vi "RtdeGetLatestOutputValues.vi"(8 "Rtde":refnum<k24>, 11 "error in":errorcluster) -> (0 "Data":T1, 3 "error out":errorcluster)   [LabVIEW 2022 SP3, in "UnderAutomation.UniversalRobots.lvlib"]
uses:
  UnderAutomation.UniversalRobots.lvlib
  C:/Users/fg/Documents/UniversalRobots.vi/LabVIEW_2023/UnderAutomation.UniversalRobots/lib/UnderAutomation.UniversalRobots.dll
  LabVIEW_2023/UnderAutomation.UniversalRobots/lib/UnderAutomation.UniversalRobots.dll
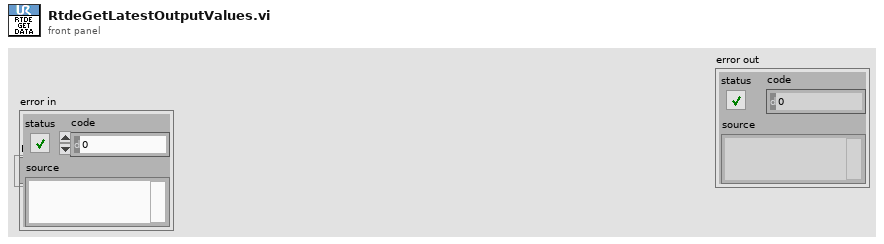
[diagram p1: front panel]
types:
  T1 = cluster{"ActualCurrent":cluster{"Base":dbl, "Elbow":dbl, "Shoulder":dbl, "Wrist1":dbl, "Wrist2":dbl, "Wrist3":dbl}, "ActualDigitalInputBits":u64, "ActualDigitalOutputBits":u64, "ActualExecutionTime":dbl, "ActualJointVoltage":cluster{"Base":dbl, "Elbow":dbl, "Shoulder":dbl, "Wrist1":dbl, "Wrist2":dbl, "Wrist3":dbl}, "ActualMainVoltage":dbl, "ActualMomentum":dbl, "ActualQ":cluster{"Base":dbl, "Elbow":dbl, "Shoulder":dbl, "Wrist1":dbl, "Wrist2":dbl, "Wrist3":dbl}, "ActualQd":cluster{"Base":dbl, "Elbow":dbl, "Shoulder":dbl, "Wrist1":dbl, "Wrist2":dbl, "Wrist3":dbl}, "ActualRobotCurrent":dbl, "ActualRobotVoltage":dbl, "ActualTcpForce":cluster{"X":dbl, "Y":dbl, "Z":dbl, "Rx":dbl, "Ry":dbl, "Rz":dbl}, "ActualTcpPose":cluster{"X":dbl, "Y":dbl, "Z":dbl, "Rx":dbl, "Ry":dbl, "Rz":dbl}, "ActualTcpSpeed":cluster{"X":dbl, "Y":dbl, "Z":dbl, "Rx":dbl, "Ry":dbl, "Rz":dbl}, "ActualToolAccelerometer":cluster{"X":dbl, "Y":dbl, "Z":dbl}, "AnalogIOTypes":u32, "ElbowPosition":cluster{"X":dbl, "Y":dbl, "Z":dbl}, "ElbowVelocity":cluster{"X":dbl, "Y":dbl, "Z":dbl}, "Euromap67_24VCurrent":dbl, "Euromap67_24VVoltage":dbl, "Euromap67InputBits":u32, "Euromap67OutputBits":u32, "FTRawWrench":cluster{"X":dbl, "Y":dbl, "Z":dbl, "Rx":dbl, "Ry":dbl, "Rz":dbl}, "InputBitRegisters":cluster{"X64":bool, "X65":bool, "X66":bool, "X67":bool, "X68":bool, "X69":bool, "X70":bool, "X71":bool, "X72":bool, "X73":bool, "X74":bool, "X75":bool, "X76":bool, "X77":bool, "X78":bool, "X79":bool, "X80":bool, "X81":bool, "X82":bool, "X83":bool, "X84":bool, "X85":bool, "X86":bool, "X87":bool, "X88":bool, "X89":bool, "X90":bool, "X91":bool, "X92":bool, "X93":bool, "X94":bool, "X95":bool, "X96":bool, "X97":bool, "X98":bool, "X99":bool, "X100":bool, "X101":bool, "X102":bool, "X103":bool, "X104":bool, "X105":bool, "X106":bool, "X107":bool, "X108":bool, "X109":bool, "X110":bool, "X111":bool, "X112":bool, "X113":bool, "X114":bool, "X115":bool, "X116":bool, "X117":bool, "X118":bool, "X119":bool, "X120":bool, "X121":bool, "X122":bool, "X123":bool, "X124":bool, "X125":bool, "X126":bool, "X127":bool}, "InputBitRegisters0To31":u32, "InputBitRegisters32To63":u32, "InputDoubleRegisters":cluster{"X0":dbl, "X1":dbl, "X2":dbl, "X3":dbl, "X4":dbl, "X5":dbl, "X6":dbl, "X7":dbl, "X8":dbl, "X9":dbl, "X10":dbl, "X11":dbl, "X12":dbl, "X13":dbl, "X14":dbl, "X15":dbl, "X16":dbl, "X17":dbl, "X18":dbl, "X19":dbl, "X20":dbl, "X21":dbl, "X22":dbl, "X23":dbl, "X24":dbl, "X25":dbl, "X26":dbl, "X27":dbl, "X28":dbl, "X29":dbl, "X30":dbl, "X31":dbl, "X32":dbl, "X33":dbl, "X34":dbl, "X35":dbl, "X36":dbl, "X37":dbl, "X38":dbl, "X39":dbl, "X40":dbl, "X41":dbl, "X42":dbl, "X43":dbl, "X44":dbl, "X45":dbl, "X46":dbl, "X47":dbl}, "InputIntRegisters":cluster{"X0":i32, "X1":i32, "X2":i32, "X3":i32, "X4":i32, "X5":i32, "X6":i32, "X7":i32, "X8":i32, "X9":i32, "X10":i32, "X11":i32, "X12":i32, "X13":i32, "X14":i32, "X15":i32, "X16":i32, "X17":i32, "X18":i32, "X19":i32, "X20":i32, "X21":i32, "X22":i32, "X23":i32, "X24":i32, "X25":i32, "X26":i32, "X27":i32, "X28":i32, "X29":i32, "X30":i32, "X31":i32, "X32":i32, "X33":i32, "X34":i32, "X35":i32, "X36":i32, "X37":i32, "X38":i32, "X39":i32, "X40":i32, "X41":i32, "X42":i32, "X43":i32, "X44":i32, "X45":i32, "X46":i32, "X47":i32}, "IOCurrent":dbl, "JointControlOutput":cluster{"Base":dbl, "Elbow":dbl, "Shoulder":dbl, "Wrist1":dbl, "Wrist2":dbl, "Wrist3":dbl}, "JointMode":cluster{"Base":i32, "Elbow":i32, "Shoulder":i32, "Wrist1":i32, "Wrist2":i32, "Wrist3":i32}, "JointTemperatures":cluster{"Base":dbl, "Elbow":dbl, "Shoulder":dbl, "Wrist1":dbl, "Wrist2":dbl, "Wrist3":dbl}, "OutputBitRegisters":cluster{"X64":bool, "X65":bool, "X66":bool, "X67":bool, "X68":bool, "X69":bool, "X70":bool, "X71":bool, "X72":bool, "X73":bool, "X74":bool, "X75":bool, "X76":bool, "X77":bool, "X78":bool, "X79":bool, "X80":bool, "X81":bool, "X82":bool, "X83":bool, "X84":bool, "X85":bool, "X86":bool, "X87":bool, "X88":bool, "X89":bool, "X90":bool, "X91":bool, "X92":bool, "X93":bool, "X94":bool, "X95":bool, "X96":bool, "X97":bool, "X98":bool, "X99":bool, "X100":bool, "X101":bool, "X102":bool, "X103":bool, "X104":bool, "X105":bool, "X106":bool, "X107":bool, "X108":bool, "X109":bool, "X110":bool, "X111":bool, "X112":bool, "X113":bool, "X114":bool, "X115":bool, "X116":bool, "X117":bool, "X118":bool, "X119":bool, "X120":bool, "X121":bool, "X122":bool, "X123":bool, "X124":bool, "X125":bool, "X126":bool, "X127":bool}, "OutputBitRegisters0To31":u32, "OutputBitRegisters32To63":u32, "OutputDoubleRegisters":cluster{"X0":dbl, "X1":dbl, "X2":dbl, "X3":dbl, "X4":dbl, "X5":dbl, "X6":dbl, "X7":dbl, "X8":dbl, "X9":dbl, "X10":dbl, "X11":dbl, "X12":dbl, "X13":dbl, "X14":dbl, "X15":dbl, "X16":dbl, "X17":dbl, "X18":dbl, "X19":dbl, "X20":dbl, "X21":dbl, "X22":dbl, "X23":dbl, "X24":dbl, "X25":dbl, "X26":dbl, "X27":dbl, "X28":dbl, "X29":dbl, "X30":dbl, "X31":dbl, "X32":dbl, "X33":dbl, "X34":dbl, "X35":dbl, "X36":dbl, "X37":dbl, "X38":dbl, "X39":dbl, "X40":dbl, "X41":dbl, "X42":dbl, "X43":dbl, "X44":dbl, "X45":dbl, "X46":dbl, "X47":dbl}, "OutputIntRegisters":cluster{"X0":i32, "X1":i32, "X2":i32, "X3":i32, "X4":i32, "X5":i32, "X6":i32, "X7":i32, "X8":i32, "X9":i32, "X10":i32, "X11":i32, "X12":i32, "X13":i32, "X14":i32, "X15":i32, "X16":i32, "X17":i32, "X18":i32, "X19":i32, "X20":i32, "X21":i32, "X22":i32, "X23":i32, "X24":i32, "X25":i32, "X26":i32, "X27":i32, "X28":i32, "X29":i32, "X30":i32, "X31":i32, "X32":i32, "X33":i32, "X34":i32, "X35":i32, "X36":i32, "X37":i32, "X38":i32, "X39":i32, "X40":i32, "X41":i32, "X42":i32, "X43":i32, "X44":i32, "X45":i32, "X46":i32, "X47":i32}, "Payload":dbl, "PayloadCOG":cluster{"X":dbl, "Y":dbl, "Z":dbl}, "PayloadInertia":cluster{"X":dbl, "Y":dbl, "Z":dbl, "Rx":dbl, "Ry":dbl, "Rz":dbl}, "RobotMode":i32, "RobotStatusBits":u32, "RuntimeState":u32, "SafetyMode":i32, "SafetyStatus":i32, "SafetyStatusBits":u32, "ScriptControlLine":u32, "SpeedScaling":dbl, "StandardAnalogInput0":dbl, "StandardAnalogInput1":dbl, "StandardAnalogOutput0":dbl, "StandardAnalogOutput1":dbl, "TargetCurrent":cluster{"Base":dbl, "Elbow":dbl, "Shoulder":dbl, "Wrist1":dbl, "Wrist2":dbl, "Wrist3":dbl}, "TargetMoment":cluster{"Base":dbl, "Elbow":dbl, "Shoulder":dbl, "Wrist1":dbl, "Wrist2":dbl, "Wrist3":dbl}, "TargetQ":cluster{"Base":dbl, "Elbow":dbl, "Shoulder":dbl, "Wrist1":dbl, "Wrist2":dbl, "Wrist3":dbl}, "TargetQd":cluster{"Base":dbl, "Elbow":dbl, "Shoulder":dbl, "Wrist1":dbl, "Wrist2":dbl, "Wrist3":dbl}, "TargetQdd":cluster{"Base":dbl, "Elbow":dbl, "Shoulder":dbl, "Wrist1":dbl, "Wrist2":dbl, "Wrist3":dbl}, "TargetSpeedFraction":dbl, "TargetTcpPose":cluster{"X":dbl, "Y":dbl, "Z":dbl, "Rx":dbl, "Ry":dbl, "Rz":dbl}, "TargetTcpSpeed":cluster{"X":dbl, "Y":dbl, "Z":dbl, "Rx":dbl, "Ry":dbl, "Rz":dbl}, "TcpForceScalar":dbl, "Timestamp":dbl, "ToolAnalogInput0":dbl, "ToolAnalogInput1":dbl, "ToolAnalogInputTypes":u32, "ToolDigitalOutput0mode":u8, "ToolDigitalOutput1Mode":u8, "ToolMode":u32, "ToolOutputCurrent":dbl, "ToolOutputMode":u8, "ToolOutputVoltage":i32, "ToolTemperature":dbl}
  T2 = cluster{"Base":dbl, "Elbow":dbl, "Shoulder":dbl, "Wrist1":dbl, "Wrist2":dbl, "Wrist3":dbl}
  T3 = cluster{"X":dbl, "Y":dbl, "Z":dbl, "Rx":dbl, "Ry":dbl, "Rz":dbl}
  T4 = cluster{"X64":bool, "X65":bool, "X66":bool, "X67":bool, "X68":bool, "X69":bool, "X70":bool, "X71":bool, "X72":bool, "X73":bool, "X74":bool, "X75":bool, "X76":bool, "X77":bool, "X78":bool, "X79":bool, "X80":bool, "X81":bool, "X82":bool, "X83":bool, "X84":bool, "X85":bool, "X86":bool, "X87":bool, "X88":bool, "X89":bool, "X90":bool, "X91":bool, "X92":bool, "X93":bool, "X94":bool, "X95":bool, "X96":bool, "X97":bool, "X98":bool, "X99":bool, "X100":bool, "X101":bool, "X102":bool, "X103":bool, "X104":bool, "X105":bool, "X106":bool, "X107":bool, "X108":bool, "X109":bool, "X110":bool, "X111":bool, "X112":bool, "X113":bool, "X114":bool, "X115":bool, "X116":bool, "X117":bool, "X118":bool, "X119":bool, "X120":bool, "X121":bool, "X122":bool, "X123":bool, "X124":bool, "X125":bool, "X126":bool, "X127":bool}
  T5 = cluster{"X0":dbl, "X1":dbl, "X2":dbl, "X3":dbl, "X4":dbl, "X5":dbl, "X6":dbl, "X7":dbl, "X8":dbl, "X9":dbl, "X10":dbl, "X11":dbl, "X12":dbl, "X13":dbl, "X14":dbl, "X15":dbl, "X16":dbl, "X17":dbl, "X18":dbl, "X19":dbl, "X20":dbl, "X21":dbl, "X22":dbl, "X23":dbl, "X24":dbl, "X25":dbl, "X26":dbl, "X27":dbl, "X28":dbl, "X29":dbl, "X30":dbl, "X31":dbl, "X32":dbl, "X33":dbl, "X34":dbl, "X35":dbl, "X36":dbl, "X37":dbl, "X38":dbl, "X39":dbl, "X40":dbl, "X41":dbl, "X42":dbl, "X43":dbl, "X44":dbl, "X45":dbl, "X46":dbl, "X47":dbl}
  T6 = cluster{"Base":i32, "Elbow":i32, "Shoulder":i32, "Wrist1":i32, "Wrist2":i32, "Wrist3":i32}
  T7 = cluster{"X0":i32, "X1":i32, "X2":i32, "X3":i32, "X4":i32, "X5":i32, "X6":i32, "X7":i32, "X8":i32, "X9":i32, "X10":i32, "X11":i32, "X12":i32, "X13":i32, "X14":i32, "X15":i32, "X16":i32, "X17":i32, "X18":i32, "X19":i32, "X20":i32, "X21":i32, "X22":i32, "X23":i32, "X24":i32, "X25":i32, "X26":i32, "X27":i32, "X28":i32, "X29":i32, "X30":i32, "X31":i32, "X32":i32, "X33":i32, "X34":i32, "X35":i32, "X36":i32, "X37":i32, "X38":i32, "X39":i32, "X40":i32, "X41":i32, "X42":i32, "X43":i32, "X44":i32, "X45":i32, "X46":i32, "X47":i32}
  T8 = cluster{cluster{"Base":dbl, "Elbow":dbl, "Shoulder":dbl, "Wrist1":dbl, "Wrist2":dbl, "Wrist3":dbl}, "ActualDigitalInputBits":u64, "ActualDigitalOutputBits":u64, "ActualExecutionTime":dbl, cluster{"Base":dbl, "Elbow":dbl, "Shoulder":dbl, "Wrist1":dbl, "Wrist2":dbl, "Wrist3":dbl}, "ActualMainVoltage":dbl, "ActualMomentum":dbl, cluster{"Base":dbl, "Elbow":dbl, "Shoulder":dbl, "Wrist1":dbl, "Wrist2":dbl, "Wrist3":dbl}, cluster{"Base":dbl, "Elbow":dbl, "Shoulder":dbl, "Wrist1":dbl, "Wrist2":dbl, "Wrist3":dbl}, "ActualRobotCurrent":dbl, "ActualRobotVoltage":dbl, cluster{"X":dbl, "Y":dbl, "Z":dbl, "Rx":dbl, "Ry":dbl, "Rz":dbl}, cluster{"X":dbl, "Y":dbl, "Z":dbl, "Rx":dbl, "Ry":dbl, "Rz":dbl}, cluster{"X":dbl, "Y":dbl, "Z":dbl, "Rx":dbl, "Ry":dbl, "Rz":dbl}, cluster{"X":dbl, "Y":dbl, "Z":dbl}, "AnalogIOTypes":u32, cluster{"X":dbl, "Y":dbl, "Z":dbl}, cluster{"X":dbl, "Y":dbl, "Z":dbl}, "Euromap67_24VCurrent":dbl, "Euromap67_24VVoltage":dbl, "Euromap67InputBits":u32, "Euromap67OutputBits":u32, cluster{"X":dbl, "Y":dbl, "Z":dbl, "Rx":dbl, "Ry":dbl, "Rz":dbl}, cluster{"X64":bool, "X65":bool, "X66":bool, "X67":bool, "X68":bool, "X69":bool, "X70":bool, "X71":bool, "X72":bool, "X73":bool, "X74":bool, "X75":bool, "X76":bool, "X77":bool, "X78":bool, "X79":bool, "X80":bool, "X81":bool, "X82":bool, "X83":bool, "X84":bool, "X85":bool, "X86":bool, "X87":bool, "X88":bool, "X89":bool, "X90":bool, "X91":bool, "X92":bool, "X93":bool, "X94":bool, "X95":bool, "X96":bool, "X97":bool, "X98":bool, "X99":bool, "X100":bool, "X101":bool, "X102":bool, "X103":bool, "X104":bool, "X105":bool, "X106":bool, "X107":bool, "X108":bool, "X109":bool, "X110":bool, "X111":bool, "X112":bool, "X113":bool, "X114":bool, "X115":bool, "X116":bool, "X117":bool, "X118":bool, "X119":bool, "X120":bool, "X121":bool, "X122":bool, "X123":bool, "X124":bool, "X125":bool, "X126":bool, "X127":bool}, "InputBitRegisters0To31":u32, "InputBitRegisters32To63":u32, cluster{"X0":dbl, "X1":dbl, "X2":dbl, "X3":dbl, "X4":dbl, "X5":dbl, "X6":dbl, "X7":dbl, "X8":dbl, "X9":dbl, "X10":dbl, "X11":dbl, "X12":dbl, "X13":dbl, "X14":dbl, "X15":dbl, "X16":dbl, "X17":dbl, "X18":dbl, "X19":dbl, "X20":dbl, "X21":dbl, "X22":dbl, "X23":dbl, "X24":dbl, "X25":dbl, "X26":dbl, "X27":dbl, "X28":dbl, "X29":dbl, "X30":dbl, "X31":dbl, "X32":dbl, "X33":dbl, "X34":dbl, "X35":dbl, "X36":dbl, "X37":dbl, "X38":dbl, "X39":dbl, "X40":dbl, "X41":dbl, "X42":dbl, "X43":dbl, "X44":dbl, "X45":dbl, "X46":dbl, "X47":dbl}, cluster{"X0":i32, "X1":i32, "X2":i32, "X3":i32, "X4":i32, "X5":i32, "X6":i32, "X7":i32, "X8":i32, "X9":i32, "X10":i32, "X11":i32, "X12":i32, "X13":i32, "X14":i32, "X15":i32, "X16":i32, "X17":i32, "X18":i32, "X19":i32, "X20":i32, "X21":i32, "X22":i32, "X23":i32, "X24":i32, "X25":i32, "X26":i32, "X27":i32, "X28":i32, "X29":i32, "X30":i32, "X31":i32, "X32":i32, "X33":i32, "X34":i32, "X35":i32, "X36":i32, "X37":i32, "X38":i32, "X39":i32, "X40":i32, "X41":i32, "X42":i32, "X43":i32, "X44":i32, "X45":i32, "X46":i32, "X47":i32}, "IOCurrent":dbl, cluster{"Base":dbl, "Elbow":dbl, "Shoulder":dbl, "Wrist1":dbl, "Wrist2":dbl, "Wrist3":dbl}, cluster{"Base":i32, "Elbow":i32, "Shoulder":i32, "Wrist1":i32, "Wrist2":i32, "Wrist3":i32}, cluster{"Base":dbl, "Elbow":dbl, "Shoulder":dbl, "Wrist1":dbl, "Wrist2":dbl, "Wrist3":dbl}, cluster{"X64":bool, "X65":bool, "X66":bool, "X67":bool, "X68":bool, "X69":bool, "X70":bool, "X71":bool, "X72":bool, "X73":bool, "X74":bool, "X75":bool, "X76":bool, "X77":bool, "X78":bool, "X79":bool, "X80":bool, "X81":bool, "X82":bool, "X83":bool, "X84":bool, "X85":bool, "X86":bool, "X87":bool, "X88":bool, "X89":bool, "X90":bool, "X91":bool, "X92":bool, "X93":bool, "X94":bool, "X95":bool, "X96":bool, "X97":bool, "X98":bool, "X99":bool, "X100":bool, "X101":bool, "X102":bool, "X103":bool, "X104":bool, "X105":bool, "X106":bool, "X107":bool, "X108":bool, "X109":bool, "X110":bool, "X111":bool, "X112":bool, "X113":bool, "X114":bool, "X115":bool, "X116":bool, "X117":bool, "X118":bool, "X119":bool, "X120":bool, "X121":bool, "X122":bool, "X123":bool, "X124":bool, "X125":bool, "X126":bool, "X127":bool}, "OutputBitRegisters0To31":u32, "OutputBitRegisters32To63":u32, cluster{"X0":dbl, "X1":dbl, "X2":dbl, "X3":dbl, "X4":dbl, "X5":dbl, "X6":dbl, "X7":dbl, "X8":dbl, "X9":dbl, "X10":dbl, "X11":dbl, "X12":dbl, "X13":dbl, "X14":dbl, "X15":dbl, "X16":dbl, "X17":dbl, "X18":dbl, "X19":dbl, "X20":dbl, "X21":dbl, "X22":dbl, "X23":dbl, "X24":dbl, "X25":dbl, "X26":dbl, "X27":dbl, "X28":dbl, "X29":dbl, "X30":dbl, "X31":dbl, "X32":dbl, "X33":dbl, "X34":dbl, "X35":dbl, "X36":dbl, "X37":dbl, "X38":dbl, "X39":dbl, "X40":dbl, "X41":dbl, "X42":dbl, "X43":dbl, "X44":dbl, "X45":dbl, "X46":dbl, "X47":dbl}, cluster{"X0":i32, "X1":i32, "X2":i32, "X3":i32, "X4":i32, "X5":i32, "X6":i32, "X7":i32, "X8":i32, "X9":i32, "X10":i32, "X11":i32, "X12":i32, "X13":i32, "X14":i32, "X15":i32, "X16":i32, "X17":i32, "X18":i32, "X19":i32, "X20":i32, "X21":i32, "X22":i32, "X23":i32, "X24":i32, "X25":i32, "X26":i32, "X27":i32, "X28":i32, "X29":i32, "X30":i32, "X31":i32, "X32":i32, "X33":i32, "X34":i32, "X35":i32, "X36":i32, "X37":i32, "X38":i32, "X39":i32, "X40":i32, "X41":i32, "X42":i32, "X43":i32, "X44":i32, "X45":i32, "X46":i32, "X47":i32}, "Payload":dbl, cluster{"X":dbl, "Y":dbl, "Z":dbl}, cluster{"X":dbl, "Y":dbl, "Z":dbl, "Rx":dbl, "Ry":dbl, "Rz":dbl}, "RobotMode":i32, "RobotStatusBits":u32, "RuntimeState":u32, "SafetyMode":i32, "SafetyStatus":i32, "SafetyStatusBits":u32, "ScriptControlLine":u32, "SpeedScaling":dbl, "StandardAnalogInput0":dbl, "StandardAnalogInput1":dbl, "StandardAnalogOutput0":dbl, "StandardAnalogOutput1":dbl, cluster{"Base":dbl, "Elbow":dbl, "Shoulder":dbl, "Wrist1":dbl, "Wrist2":dbl, "Wrist3":dbl}, cluster{"Base":dbl, "Elbow":dbl, "Shoulder":dbl, "Wrist1":dbl, "Wrist2":dbl, "Wrist3":dbl}, cluster{"Base":dbl, "Elbow":dbl, "Shoulder":dbl, "Wrist1":dbl, "Wrist2":dbl, "Wrist3":dbl}, cluster{"Base":dbl, "Elbow":dbl, "Shoulder":dbl, "Wrist1":dbl, "Wrist2":dbl, "Wrist3":dbl}, cluster{"Base":dbl, "Elbow":dbl, "Shoulder":dbl, "Wrist1":dbl, "Wrist2":dbl, "Wrist3":dbl}, "TargetSpeedFraction":dbl, cluster{"X":dbl, "Y":dbl, "Z":dbl, "Rx":dbl, "Ry":dbl, "Rz":dbl}, cluster{"X":dbl, "Y":dbl, "Z":dbl, "Rx":dbl, "Ry":dbl, "Rz":dbl}, "TcpForceScalar":dbl, "Timestamp":dbl, "ToolAnalogInput0":dbl, "ToolAnalogInput1":dbl, "ToolAnalogInputTypes":u32, "ToolDigitalOutput0mode":u8, "ToolDigitalOutput1Mode":u8, "ToolMode":u32, "ToolOutputCurrent":dbl, "ToolOutputMode":u8, "ToolOutputVoltage":i32, "ToolTemperature":dbl}
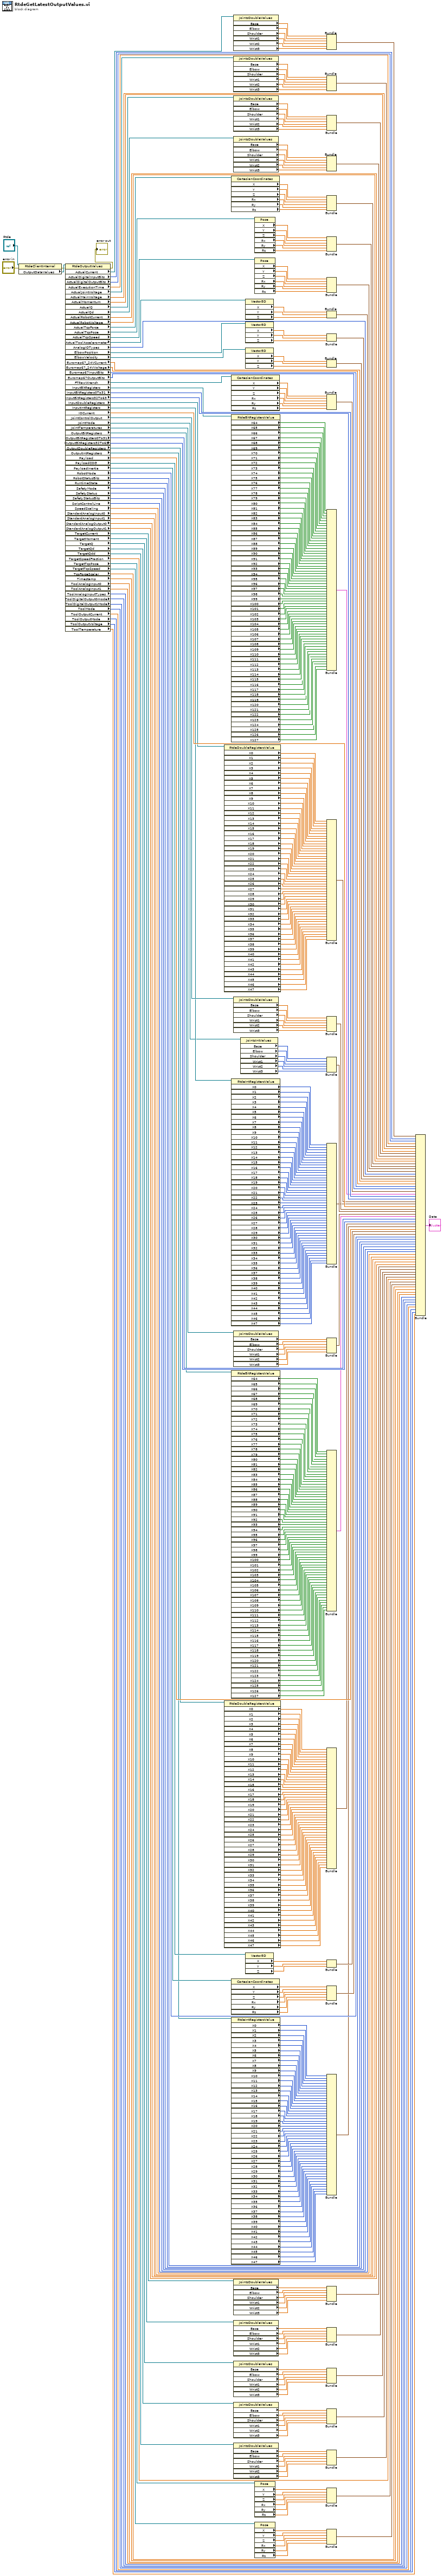
[diagram p0: block diagram]
diagram:
  n1 = property class="RtdeClientInternal"(reference="Rtde", error in="error in") -> (error out=w1:errorcluster, "OutputDataValues"=w2:refnum<k24>)  [unwired: 1 out]
  n2 = property on="Property Node" class="RtdeOutputValues"(reference=w2, error in=w1) -> (error out=→"error out":errorcluster, "ActualCurrent"=w4:refnum<k24>, "ActualDigitalInputBits"=w126:u64, "ActualDigitalOutputBits"=w127:u64, "ActualExecutionTime"=w128:dbl, "ActualJointVoltage"=w11:refnum<k24>, "ActualMainVoltage"=w130:dbl, "ActualMomentum"=w131:dbl, "ActualQ"=w83:refnum<k24>, "ActualQd"=w90:refnum<k24>, "ActualRobotCurrent"=w134:dbl, "ActualRobotVoltage"=w135:dbl, "ActualTcpForce"=w149:refnum<k24>, "ActualTcpPose"=w136:refnum<k24>, "ActualTcpSpeed"=w158:refnum<k24>, "ActualToolAccelerometer"=w160:refnum<k24>, "AnalogIOTypes"=w165:u32, "ElbowPosition"=w166:refnum<k24>, "ElbowVelocity"=w171:refnum<k24>, "Euromap67_24VCurrent"=w176:dbl, "Euromap67_24VVoltage"=w177:dbl, "Euromap67InputBits"=w178:u32, "Euromap67OutputBits"=w179:u32, "FTRawWrench"=w186:refnum<k24>, "InputBitRegisters"=w252:refnum<k24>, "InputBitRegisters0To31"=w304:u32, "InputBitRegisters32To63"=w303:u32, "InputDoubleRegisters"=w254:refnum<k24>, "InputIntRegisters"=w354:refnum<k24>, "IOCurrent"=w356:dbl, "JointControlOutput"=w363:refnum<k24>, "JointMode"=w97:refnum<k24>, "JointTemperatures"=w372:refnum<k24>, "OutputBitRegisters"=w12:refnum<k24>, "OutputBitRegisters0To31"=w375:u32, "OutputBitRegisters32To63"=w376:u32, "OutputDoubleRegisters"=w425:refnum<k24>, "OutputIntRegisters"=w475:refnum<k24>, "Payload"=w481:dbl, "PayloadCOG"=w480:refnum<k24>, "PayloadInertia"=w489:refnum<k24>, "RobotMode"=w491:i32, "RobotStatusBits"=w492:u32, "RuntimeState"=w493:u32, "SafetyMode"=w494:i32, "SafetyStatus"=w495:i32, "SafetyStatusBits"=w496:u32, "ScriptControlLine"=w497:u32, "SpeedScaling"=w498:dbl, "StandardAnalogInput0"=w499:dbl, "StandardAnalogInput1"=w500:dbl, "StandardAnalogOutput0"=w501:dbl, "StandardAnalogOutput1"=w502:dbl, "TargetCurrent"=w515:refnum<k24>, "TargetMoment"=w516:refnum<k24>, "TargetQ"=w122:refnum<k24>, "TargetQd"=w123:refnum<k24>, "TargetQdd"=w124:refnum<k24>, "TargetSpeedFraction"=w522:dbl, "TargetTcpPose"=w535:refnum<k24>, "TargetTcpSpeed"=w536:refnum<k24>, "TcpForceScalar"=w539:dbl, "Timestamp"=w540:dbl, "ToolAnalogInput0"=w541:dbl, "ToolAnalogInput1"=w542:dbl, "ToolAnalogInputTypes"=w543:u32, "ToolDigitalOutput0mode"=w544:u8, "ToolDigitalOutput1Mode"=w545:u8, "ToolMode"=w546:u32, "ToolOutputCurrent"=w547:dbl, "ToolOutputMode"=w548:u8, "ToolOutputVoltage"=w549:i32, "ToolTemperature"=w550:dbl)  [unwired: 1 out]
  n3 = property class="RtdeDoubleRegistersValue"(reference=w254) -> ("X0"=w255:dbl, "X1"=w256:dbl, "X2"=w257:dbl, "X3"=w258:dbl, "X4"=w259:dbl, "X5"=w260:dbl, "X6"=w261:dbl, "X7"=w262:dbl, "X8"=w263:dbl, "X9"=w264:dbl, "X10"=w265:dbl, "X11"=w266:dbl, "X12"=w267:dbl, "X13"=w268:dbl, "X14"=w269:dbl, "X15"=w270:dbl, "X16"=w271:dbl, "X17"=w272:dbl, "X18"=w273:dbl, "X19"=w274:dbl, "X20"=w275:dbl, "X21"=w276:dbl, "X22"=w277:dbl, "X23"=w278:dbl, "X24"=w279:dbl, "X25"=w280:dbl, "X26"=w281:dbl, "X27"=w282:dbl, "X28"=w283:dbl, "X29"=w284:dbl, "X30"=w285:dbl, "X31"=w286:dbl, "X32"=w287:dbl, "X33"=w288:dbl, "X34"=w289:dbl, "X35"=w290:dbl, "X36"=w291:dbl, "X37"=w292:dbl, "X38"=w293:dbl, "X39"=w294:dbl, "X40"=w295:dbl, "X41"=w296:dbl, "X42"=w297:dbl, "X43"=w298:dbl, "X44"=w299:dbl, "X45"=w300:dbl, "X46"=w301:dbl, "X47"=w302:dbl)  [unwired: 1 in, 2 out]
  n4 = property class="RtdeDoubleRegistersValue"(reference=w425) -> ("X0"=w377:dbl, "X1"=w378:dbl, "X2"=w379:dbl, "X3"=w380:dbl, "X4"=w381:dbl, "X5"=w382:dbl, "X6"=w383:dbl, "X7"=w384:dbl, "X8"=w385:dbl, "X9"=w386:dbl, "X10"=w387:dbl, "X11"=w388:dbl, "X12"=w389:dbl, "X13"=w390:dbl, "X14"=w391:dbl, "X15"=w392:dbl, "X16"=w393:dbl, "X17"=w394:dbl, "X18"=w395:dbl, "X19"=w396:dbl, "X20"=w397:dbl, "X21"=w398:dbl, "X22"=w399:dbl, "X23"=w400:dbl, "X24"=w401:dbl, "X25"=w402:dbl, "X26"=w403:dbl, "X27"=w404:dbl, "X28"=w405:dbl, "X29"=w406:dbl, "X30"=w407:dbl, "X31"=w408:dbl, "X32"=w409:dbl, "X33"=w410:dbl, "X34"=w411:dbl, "X35"=w412:dbl, "X36"=w413:dbl, "X37"=w414:dbl, "X38"=w415:dbl, "X39"=w416:dbl, "X40"=w417:dbl, "X41"=w418:dbl, "X42"=w419:dbl, "X43"=w420:dbl, "X44"=w421:dbl, "X45"=w422:dbl, "X46"=w423:dbl, "X47"=w424:dbl)  [unwired: 1 in, 2 out]
  n5 = property class="CartesianCoordinates"(reference=w149) -> ("X"=w148:dbl, "Y"=w147:dbl, "Z"=w146:dbl, "Rx"=w145:dbl, "Ry"=w144:dbl, "Rz"=w143:dbl)  [unwired: 1 in, 2 out]
  n6 = property class="CartesianCoordinates"(reference=w186) -> ("X"=w180:dbl, "Y"=w181:dbl, "Z"=w182:dbl, "Rx"=w183:dbl, "Ry"=w184:dbl, "Rz"=w185:dbl)  [unwired: 1 in, 2 out]
  n7 = property class="CartesianCoordinates"(reference=w489) -> ("X"=w483:dbl, "Y"=w484:dbl, "Z"=w485:dbl, "Rx"=w486:dbl, "Ry"=w487:dbl, "Rz"=w488:dbl)  [unwired: 1 in, 2 out]
  n8 = property class="RtdeBitRegistersValue"(reference=w252) -> ("X64"=w251:bool, "X65"=w250:bool, "X66"=w249:bool, "X67"=w248:bool, "X68"=w247:bool, "X69"=w246:bool, "X70"=w245:bool, "X71"=w244:bool, "X72"=w243:bool, "X73"=w242:bool, "X74"=w241:bool, "X75"=w240:bool, "X76"=w239:bool, "X77"=w238:bool, "X78"=w237:bool, "X79"=w236:bool, "X80"=w235:bool, "X81"=w234:bool, "X82"=w233:bool, "X83"=w232:bool, "X84"=w231:bool, "X85"=w230:bool, "X86"=w229:bool, "X87"=w228:bool, "X88"=w227:bool, "X89"=w226:bool, "X90"=w225:bool, "X91"=w224:bool, "X92"=w223:bool, "X93"=w222:bool, "X94"=w221:bool, "X95"=w220:bool, "X96"=w219:bool, "X97"=w218:bool, "X98"=w217:bool, "X99"=w216:bool, "X100"=w215:bool, "X101"=w214:bool, "X102"=w213:bool, "X103"=w212:bool, "X104"=w211:bool, "X105"=w210:bool, "X106"=w209:bool, "X107"=w208:bool, "X108"=w207:bool, "X109"=w206:bool, "X110"=w205:bool, "X111"=w204:bool, "X112"=w203:bool, "X113"=w202:bool, "X114"=w201:bool, "X115"=w200:bool, "X116"=w199:bool, "X117"=w198:bool, "X118"=w197:bool, "X119"=w196:bool, "X120"=w195:bool, "X121"=w194:bool, "X122"=w193:bool, "X123"=w192:bool, "X124"=w191:bool, "X125"=w190:bool, "X126"=w189:bool, "X127"=w188:bool)  [unwired: 1 in, 2 out]
  n9 = property class="RtdeIntRegistersValue"(reference=w354) -> ("X0"=w306:i32, "X1"=w307:i32, "X2"=w308:i32, "X3"=w309:i32, "X4"=w310:i32, "X5"=w311:i32, "X6"=w312:i32, "X7"=w313:i32, "X8"=w314:i32, "X9"=w315:i32, "X10"=w316:i32, "X11"=w317:i32, "X12"=w318:i32, "X13"=w319:i32, "X14"=w320:i32, "X15"=w321:i32, "X16"=w322:i32, "X17"=w323:i32, "X18"=w324:i32, "X19"=w325:i32, "X20"=w326:i32, "X21"=w327:i32, "X22"=w328:i32, "X23"=w329:i32, "X24"=w330:i32, "X25"=w331:i32, "X26"=w332:i32, "X27"=w333:i32, "X28"=w334:i32, "X29"=w335:i32, "X30"=w336:i32, "X31"=w337:i32, "X32"=w338:i32, "X33"=w339:i32, "X34"=w340:i32, "X35"=w341:i32, "X36"=w342:i32, "X37"=w343:i32, "X38"=w344:i32, "X39"=w345:i32, "X40"=w346:i32, "X41"=w347:i32, "X42"=w348:i32, "X43"=w349:i32, "X44"=w350:i32, "X45"=w351:i32, "X46"=w352:i32, "X47"=w353:i32)  [unwired: 1 in, 2 out]
  n10 = property class="RtdeBitRegistersValue"(reference=w12) -> ("X64"=w13:bool, "X65"=w14:bool, "X66"=w15:bool, "X67"=w16:bool, "X68"=w17:bool, "X69"=w18:bool, "X70"=w19:bool, "X71"=w20:bool, "X72"=w21:bool, "X73"=w22:bool, "X74"=w23:bool, "X75"=w24:bool, "X76"=w25:bool, "X77"=w26:bool, "X78"=w27:bool, "X79"=w28:bool, "X80"=w29:bool, "X81"=w30:bool, "X82"=w31:bool, "X83"=w32:bool, "X84"=w33:bool, "X85"=w34:bool, "X86"=w35:bool, "X87"=w36:bool, "X88"=w37:bool, "X89"=w38:bool, "X90"=w39:bool, "X91"=w40:bool, "X92"=w41:bool, "X93"=w42:bool, "X94"=w43:bool, "X95"=w44:bool, "X96"=w45:bool, "X97"=w46:bool, "X98"=w47:bool, "X99"=w48:bool, "X100"=w49:bool, "X101"=w50:bool, "X102"=w51:bool, "X103"=w52:bool, "X104"=w53:bool, "X105"=w54:bool, "X106"=w55:bool, "X107"=w56:bool, "X108"=w57:bool, "X109"=w58:bool, "X110"=w59:bool, "X111"=w60:bool, "X112"=w61:bool, "X113"=w62:bool, "X114"=w63:bool, "X115"=w64:bool, "X116"=w65:bool, "X117"=w66:bool, "X118"=w67:bool, "X119"=w68:bool, "X120"=w69:bool, "X121"=w70:bool, "X122"=w71:bool, "X123"=w72:bool, "X124"=w73:bool, "X125"=w74:bool, "X126"=w75:bool, "X127"=w76:bool)  [unwired: 1 in, 2 out]
  n11 = property class="RtdeIntRegistersValue"(reference=w475) -> ("X0"=w474:i32, "X1"=w473:i32, "X2"=w472:i32, "X3"=w471:i32, "X4"=w470:i32, "X5"=w469:i32, "X6"=w468:i32, "X7"=w467:i32, "X8"=w466:i32, "X9"=w465:i32, "X10"=w464:i32, "X11"=w463:i32, "X12"=w462:i32, "X13"=w461:i32, "X14"=w460:i32, "X15"=w459:i32, "X16"=w458:i32, "X17"=w457:i32, "X18"=w456:i32, "X19"=w455:i32, "X20"=w454:i32, "X21"=w453:i32, "X22"=w452:i32, "X23"=w451:i32, "X24"=w450:i32, "X25"=w449:i32, "X26"=w448:i32, "X27"=w447:i32, "X28"=w446:i32, "X29"=w445:i32, "X30"=w444:i32, "X31"=w443:i32, "X32"=w442:i32, "X33"=w441:i32, "X34"=w440:i32, "X35"=w439:i32, "X36"=w438:i32, "X37"=w437:i32, "X38"=w436:i32, "X39"=w435:i32, "X40"=w434:i32, "X41"=w433:i32, "X42"=w432:i32, "X43"=w431:i32, "X44"=w430:i32, "X45"=w429:i32, "X46"=w428:i32, "X47"=w427:i32)  [unwired: 1 in, 2 out]
  n12 = property class="JointsDoubleValues"(reference=w4) -> ("Base"=w5:dbl, "Elbow"=w6:dbl, "Shoulder"=w7:dbl, "Wrist1"=w8:dbl, "Wrist2"=w9:dbl, "Wrist3"=w10:dbl)  [unwired: 1 in, 2 out]
  n13 = property class="JointsDoubleValues"(reference=w11) -> ("Base"=w91:dbl, "Elbow"=w92:dbl, "Shoulder"=w93:dbl, "Wrist1"=w94:dbl, "Wrist2"=w95:dbl, "Wrist3"=w96:dbl)  [unwired: 1 in, 2 out]
  n14 = property class="JointsDoubleValues"(reference=w83) -> ("Base"=w77:dbl, "Elbow"=w78:dbl, "Shoulder"=w79:dbl, "Wrist1"=w80:dbl, "Wrist2"=w81:dbl, "Wrist3"=w82:dbl)  [unwired: 1 in, 2 out]
  n15 = property class="JointsDoubleValues"(reference=w90) -> ("Base"=w84:dbl, "Elbow"=w85:dbl, "Shoulder"=w86:dbl, "Wrist1"=w87:dbl, "Wrist2"=w88:dbl, "Wrist3"=w89:dbl)  [unwired: 1 in, 2 out]
  n16 = property class="JointsDoubleValues"(reference=w363) -> ("Base"=w357:dbl, "Elbow"=w358:dbl, "Shoulder"=w359:dbl, "Wrist1"=w360:dbl, "Wrist2"=w361:dbl, "Wrist3"=w362:dbl)  [unwired: 1 in, 2 out]
  n17 = property class="JointsDoubleValues"(reference=w372) -> ("Base"=w371:dbl, "Elbow"=w370:dbl, "Shoulder"=w369:dbl, "Wrist1"=w368:dbl, "Wrist2"=w367:dbl, "Wrist3"=w366:dbl)  [unwired: 1 in, 2 out]
  n18 = property class="JointsDoubleValues"(reference=w515) -> ("Base"=w509:dbl, "Elbow"=w510:dbl, "Shoulder"=w511:dbl, "Wrist1"=w512:dbl, "Wrist2"=w513:dbl, "Wrist3"=w514:dbl)  [unwired: 1 in, 2 out]
  n19 = property class="JointsDoubleValues"(reference=w516) -> ("Base"=w508:dbl, "Elbow"=w507:dbl, "Shoulder"=w506:dbl, "Wrist1"=w505:dbl, "Wrist2"=w504:dbl, "Wrist3"=w503:dbl)  [unwired: 1 in, 2 out]
  n20 = property class="JointsDoubleValues"(reference=w122) -> ("Base"=w104:dbl, "Elbow"=w105:dbl, "Shoulder"=w106:dbl, "Wrist1"=w107:dbl, "Wrist2"=w108:dbl, "Wrist3"=w109:dbl)  [unwired: 1 in, 2 out]
  n21 = property class="JointsDoubleValues"(reference=w123) -> ("Base"=w110:dbl, "Elbow"=w111:dbl, "Shoulder"=w112:dbl, "Wrist1"=w113:dbl, "Wrist2"=w114:dbl, "Wrist3"=w115:dbl)  [unwired: 1 in, 2 out]
  n22 = property class="JointsDoubleValues"(reference=w124) -> ("Base"=w116:dbl, "Elbow"=w117:dbl, "Shoulder"=w118:dbl, "Wrist1"=w119:dbl, "Wrist2"=w120:dbl, "Wrist3"=w121:dbl)  [unwired: 1 in, 2 out]
  n23 = property class="JointsIntValues"(reference=w97) -> ("Base"=w98:i32, "Elbow"=w99:i32, "Shoulder"=w100:i32, "Wrist1"=w101:i32, "Wrist2"=w102:i32, "Wrist3"=w103:i32)  [unwired: 1 in, 2 out]
  n24 = property class="Vector3D"(reference=w160) -> ("X"=w161:dbl, "Y"=w162:dbl, "Z"=w163:dbl)  [unwired: 1 in, 2 out]
  n25 = property class="Vector3D"(reference=w166) -> ("X"=w167:dbl, "Y"=w168:dbl, "Z"=w169:dbl)  [unwired: 1 in, 2 out]
  n26 = property class="Vector3D"(reference=w171) -> ("X"=w172:dbl, "Y"=w173:dbl, "Z"=w174:dbl)  [unwired: 1 in, 2 out]
  n27 = property class="Vector3D"(reference=w480) -> ("X"=w477:dbl, "Y"=w478:dbl, "Z"=w479:dbl)  [unwired: 1 in, 2 out]
  n28 = property class="Pose"(reference=w136) -> ("X"=w137:dbl, "Y"=w138:dbl, "Z"=w139:dbl, "Rx"=w140:dbl, "Ry"=w141:dbl, "Rz"=w142:dbl)  [unwired: 1 in, 2 out]
  n29 = property class="Pose"(reference=w158) -> ("X"=w152:dbl, "Y"=w153:dbl, "Z"=w154:dbl, "Rx"=w155:dbl, "Ry"=w156:dbl, "Rz"=w157:dbl)  [unwired: 1 in, 2 out]
  n30 = property class="Pose"(reference=w535) -> ("X"=w523:dbl, "Y"=w524:dbl, "Z"=w525:dbl, "Rx"=w526:dbl, "Ry"=w527:dbl, "Rz"=w528:dbl)  [unwired: 1 in, 2 out]
  n31 = property class="Pose"(reference=w536) -> ("X"=w529:dbl, "Y"=w530:dbl, "Z"=w531:dbl, "Rx"=w532:dbl, "Ry"=w533:dbl, "Rz"=w534:dbl)  [unwired: 1 in, 2 out]
  n32 = Bundle("Base"=w5, "Elbow"=w6, "Shoulder"=w7, "Wrist1"=w8, "Wrist2"=w9, "Wrist3"=w10) -> (w125:T2)  [unwired: 1 in]
  n33 = Bundle("Base"=w91, "Elbow"=w92, "Shoulder"=w93, "Wrist1"=w94, "Wrist2"=w95, "Wrist3"=w96) -> (w129:T2)  [unwired: 1 in]
  n34 = Bundle("Base"=w77, "Elbow"=w78, "Shoulder"=w79, "Wrist1"=w80, "Wrist2"=w81, "Wrist3"=w82) -> (w132:T2)  [unwired: 1 in]
  n35 = Bundle("Base"=w84, "Elbow"=w85, "Shoulder"=w86, "Wrist1"=w87, "Wrist2"=w88, "Wrist3"=w89) -> (w133:T2)  [unwired: 1 in]
  n36 = Bundle("X"=w148, "Y"=w147, "Z"=w146, "Rx"=w145, "Ry"=w144, "Rz"=w143) -> (w150:T3)  [unwired: 1 in]
  n37 = Bundle("X"=w137, "Y"=w138, "Z"=w139, "Rx"=w140, "Ry"=w141, "Rz"=w142) -> (w151:T3)  [unwired: 1 in]
  n38 = Bundle("X"=w152, "Y"=w153, "Z"=w154, "Rx"=w155, "Ry"=w156, "Rz"=w157) -> (w159:T3)  [unwired: 1 in]
  n39 = Bundle("X"=w161, "Y"=w162, "Z"=w163) -> (w164:cluster{"X":dbl, "Y":dbl, "Z":dbl})  [unwired: 1 in]
  n40 = Bundle("X"=w167, "Y"=w168, "Z"=w169) -> (w170:cluster{"X":dbl, "Y":dbl, "Z":dbl})  [unwired: 1 in]
  n41 = Bundle("X"=w172, "Y"=w173, "Z"=w174) -> (w175:cluster{"X":dbl, "Y":dbl, "Z":dbl})  [unwired: 1 in]
  n42 = Bundle("X"=w180, "Y"=w181, "Z"=w182, "Rx"=w183, "Ry"=w184, "Rz"=w185) -> (w187:T3)  [unwired: 1 in]
  n43 = Bundle("X64"=w251, "X65"=w250, "X66"=w249, "X67"=w248, "X68"=w247, "X69"=w246, "X70"=w245, "X71"=w244, "X72"=w243, "X73"=w242, "X74"=w241, "X75"=w240, "X76"=w239, "X77"=w238, "X78"=w237, "X79"=w236, "X80"=w235, "X81"=w234, "X82"=w233, "X83"=w232, "X84"=w231, "X85"=w230, "X86"=w229, "X87"=w228, "X88"=w227, "X89"=w226, "X90"=w225, "X91"=w224, "X92"=w223, "X93"=w222, "X94"=w221, "X95"=w220, "X96"=w219, "X97"=w218, "X98"=w217, "X99"=w216, "X100"=w215, "X101"=w214, "X102"=w213, "X103"=w212, "X104"=w211, "X105"=w210, "X106"=w209, "X107"=w208, "X108"=w207, "X109"=w206, "X110"=w205, "X111"=w204, "X112"=w203, "X113"=w202, "X114"=w201, "X115"=w200, "X116"=w199, "X117"=w198, "X118"=w197, "X119"=w196, "X120"=w195, "X121"=w194, "X122"=w193, "X123"=w192, "X124"=w191, "X125"=w190, "X126"=w189, "X127"=w188) -> (w253:T4)  [unwired: 1 in]
  n44 = Bundle("X0"=w255, "X1"=w256, "X2"=w257, "X3"=w258, "X4"=w259, "X5"=w260, "X6"=w261, "X7"=w262, "X8"=w263, "X9"=w264, "X10"=w265, "X11"=w266, "X12"=w267, "X13"=w268, "X14"=w269, "X15"=w270, "X16"=w271, "X17"=w272, "X18"=w273, "X19"=w274, "X20"=w275, "X21"=w276, "X22"=w277, "X23"=w278, "X24"=w279, "X25"=w280, "X26"=w281, "X27"=w282, "X28"=w283, "X29"=w284, "X30"=w285, "X31"=w286, "X32"=w287, "X33"=w288, "X34"=w289, "X35"=w290, "X36"=w291, "X37"=w292, "X38"=w293, "X39"=w294, "X40"=w295, "X41"=w296, "X42"=w297, "X43"=w298, "X44"=w299, "X45"=w300, "X46"=w301, "X47"=w302) -> (w305:T5)  [unwired: 1 in]
  n45 = Bundle("Base"=w357, "Elbow"=w358, "Shoulder"=w359, "Wrist1"=w360, "Wrist2"=w361, "Wrist3"=w362) -> (w364:T2)  [unwired: 1 in]
  n46 = Bundle("Base"=w98, "Elbow"=w99, "Shoulder"=w100, "Wrist1"=w101, "Wrist2"=w102, "Wrist3"=w103) -> (w365:T6)  [unwired: 1 in]
  n47 = Bundle("X0"=w306, "X1"=w307, "X2"=w308, "X3"=w309, "X4"=w310, "X5"=w311, "X6"=w312, "X7"=w313, "X8"=w314, "X9"=w315, "X10"=w316, "X11"=w317, "X12"=w318, "X13"=w319, "X14"=w320, "X15"=w321, "X16"=w322, "X17"=w323, "X18"=w324, "X19"=w325, "X20"=w326, "X21"=w327, "X22"=w328, "X23"=w329, "X24"=w330, "X25"=w331, "X26"=w332, "X27"=w333, "X28"=w334, "X29"=w335, "X30"=w336, "X31"=w337, "X32"=w338, "X33"=w339, "X34"=w340, "X35"=w341, "X36"=w342, "X37"=w343, "X38"=w344, "X39"=w345, "X40"=w346, "X41"=w347, "X42"=w348, "X43"=w349, "X44"=w350, "X45"=w351, "X46"=w352, "X47"=w353) -> (w355:T7)  [unwired: 1 in]
  n48 = Bundle("Base"=w371, "Elbow"=w370, "Shoulder"=w369, "Wrist1"=w368, "Wrist2"=w367, "Wrist3"=w366) -> (w373:T2)  [unwired: 1 in]
  n49 = Bundle("X64"=w13, "X65"=w14, "X66"=w15, "X67"=w16, "X68"=w17, "X69"=w18, "X70"=w19, "X71"=w20, "X72"=w21, "X73"=w22, "X74"=w23, "X75"=w24, "X76"=w25, "X77"=w26, "X78"=w27, "X79"=w28, "X80"=w29, "X81"=w30, "X82"=w31, "X83"=w32, "X84"=w33, "X85"=w34, "X86"=w35, "X87"=w36, "X88"=w37, "X89"=w38, "X90"=w39, "X91"=w40, "X92"=w41, "X93"=w42, "X94"=w43, "X95"=w44, "X96"=w45, "X97"=w46, "X98"=w47, "X99"=w48, "X100"=w49, "X101"=w50, "X102"=w51, "X103"=w52, "X104"=w53, "X105"=w54, "X106"=w55, "X107"=w56, "X108"=w57, "X109"=w58, "X110"=w59, "X111"=w60, "X112"=w61, "X113"=w62, "X114"=w63, "X115"=w64, "X116"=w65, "X117"=w66, "X118"=w67, "X119"=w68, "X120"=w69, "X121"=w70, "X122"=w71, "X123"=w72, "X124"=w73, "X125"=w74, "X126"=w75, "X127"=w76) -> (w374:T4)  [unwired: 1 in]
  n50 = Bundle("X0"=w377, "X1"=w378, "X2"=w379, "X3"=w380, "X4"=w381, "X5"=w382, "X6"=w383, "X7"=w384, "X8"=w385, "X9"=w386, "X10"=w387, "X11"=w388, "X12"=w389, "X13"=w390, "X14"=w391, "X15"=w392, "X16"=w393, "X17"=w394, "X18"=w395, "X19"=w396, "X20"=w397, "X21"=w398, "X22"=w399, "X23"=w400, "X24"=w401, "X25"=w402, "X26"=w403, "X27"=w404, "X28"=w405, "X29"=w406, "X30"=w407, "X31"=w408, "X32"=w409, "X33"=w410, "X34"=w411, "X35"=w412, "X36"=w413, "X37"=w414, "X38"=w415, "X39"=w416, "X40"=w417, "X41"=w418, "X42"=w419, "X43"=w420, "X44"=w421, "X45"=w422, "X46"=w423, "X47"=w424) -> (w426:T5)  [unwired: 1 in]
  n51 = Bundle("X"=w477, "Y"=w478, "Z"=w479) -> (w482:cluster{"X":dbl, "Y":dbl, "Z":dbl})  [unwired: 1 in]
  n52 = Bundle("X"=w483, "Y"=w484, "Z"=w485, "Rx"=w486, "Ry"=w487, "Rz"=w488) -> (w490:T3)  [unwired: 1 in]
  n53 = Bundle("X0"=w474, "X1"=w473, "X2"=w472, "X3"=w471, "X4"=w470, "X5"=w469, "X6"=w468, "X7"=w467, "X8"=w466, "X9"=w465, "X10"=w464, "X11"=w463, "X12"=w462, "X13"=w461, "X14"=w460, "X15"=w459, "X16"=w458, "X17"=w457, "X18"=w456, "X19"=w455, "X20"=w454, "X21"=w453, "X22"=w452, "X23"=w451, "X24"=w450, "X25"=w449, "X26"=w448, "X27"=w447, "X28"=w446, "X29"=w445, "X30"=w444, "X31"=w443, "X32"=w442, "X33"=w441, "X34"=w440, "X35"=w439, "X36"=w438, "X37"=w437, "X38"=w436, "X39"=w435, "X40"=w434, "X41"=w433, "X42"=w432, "X43"=w431, "X44"=w430, "X45"=w429, "X46"=w428, "X47"=w427) -> (w476:T7)  [unwired: 1 in]
  n54 = Bundle("Base"=w509, "Elbow"=w510, "Shoulder"=w511, "Wrist1"=w512, "Wrist2"=w513, "Wrist3"=w514) -> (w517:T2)  [unwired: 1 in]
  n55 = Bundle("Base"=w508, "Elbow"=w507, "Shoulder"=w506, "Wrist1"=w505, "Wrist2"=w504, "Wrist3"=w503) -> (w518:T2)  [unwired: 1 in]
  n56 = Bundle("Base"=w104, "Elbow"=w105, "Shoulder"=w106, "Wrist1"=w107, "Wrist2"=w108, "Wrist3"=w109) -> (w519:T2)  [unwired: 1 in]
  n57 = Bundle("Base"=w110, "Elbow"=w111, "Shoulder"=w112, "Wrist1"=w113, "Wrist2"=w114, "Wrist3"=w115) -> (w520:T2)  [unwired: 1 in]
  n58 = Bundle("Base"=w116, "Elbow"=w117, "Shoulder"=w118, "Wrist1"=w119, "Wrist2"=w120, "Wrist3"=w121) -> (w521:T2)  [unwired: 1 in]
  n59 = Bundle("X"=w523, "Y"=w524, "Z"=w525, "Rx"=w526, "Ry"=w527, "Rz"=w528) -> (w537:T3)  [unwired: 1 in]
  n60 = Bundle("X"=w529, "Y"=w530, "Z"=w531, "Rx"=w532, "Ry"=w533, "Rz"=w534) -> (w538:T3)  [unwired: 1 in]
  n61 = Bundle(w125, "ActualDigitalInputBits"=w126, "ActualDigitalOutputBits"=w127, "ActualExecutionTime"=w128, w129, "ActualMainVoltage"=w130, "ActualMomentum"=w131, w132, w133, "ActualRobotCurrent"=w134, "ActualRobotVoltage"=w135, w150, w151, w159, w164, "AnalogIOTypes"=w165, w170, w175, "Euromap67_24VCurrent"=w176, "Euromap67_24VVoltage"=w177, "Euromap67InputBits"=w178, "Euromap67OutputBits"=w179, w187, w253, "InputBitRegisters0To31"=w304, "InputBitRegisters32To63"=w303, w305, w355, "IOCurrent"=w356, w364, w365, w373, w374, "OutputBitRegisters0To31"=w375, "OutputBitRegisters32To63"=w376, w426, w476, "Payload"=w481, w482, w490, "RobotMode"=w491, "RobotStatusBits"=w492, "RuntimeState"=w493, "SafetyMode"=w494, "SafetyStatus"=w495, "SafetyStatusBits"=w496, "ScriptControlLine"=w497, "SpeedScaling"=w498, "StandardAnalogInput0"=w499, "StandardAnalogInput1"=w500, "StandardAnalogOutput0"=w501, "StandardAnalogOutput1"=w502, w517, w518, w519, w520, w521, "TargetSpeedFraction"=w522, w537, w538, "TcpForceScalar"=w539, "Timestamp"=w540, "ToolAnalogInput0"=w541, "ToolAnalogInput1"=w542, "ToolAnalogInputTypes"=w543, "ToolDigitalOutput0mode"=w544, "ToolDigitalOutput1Mode"=w545, "ToolMode"=w546, "ToolOutputCurrent"=w547, "ToolOutputMode"=w548, "ToolOutputVoltage"=w549, "ToolTemperature"=w550) -> (→"Data":T8)  [unwired: 1 in]
